vi "FGUDP.vi"(5 "Port":u16=5502, 7 "Remote Host":string="10.0.22.163", 8 "Error In":errorcluster, 10 "Data String In":string, 11 "UDP State":T1) -> (0 "error out":errorcluster, 2 "Data String Out":string)   [LabVIEW 2010, in "Flight Gear Data Custom Device.lvlib"]
uses:
  Flight Gear Data Custom Device.lvlib
  FlightGearState.ctl
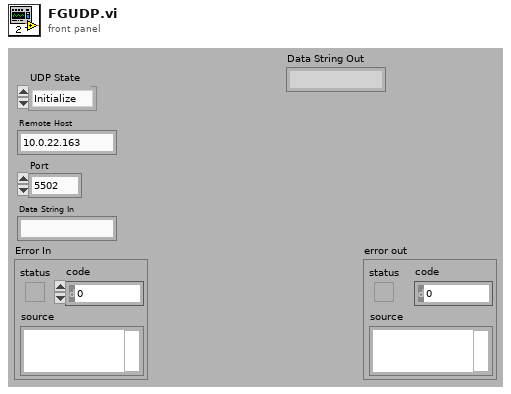
[diagram p1: front panel]
types:
  T1 = typedef "Flight Gear Data Custom Device.lvlib/FlightGearState.ctl" = enum16{"Initialize", "Read", "Write", "Close"}
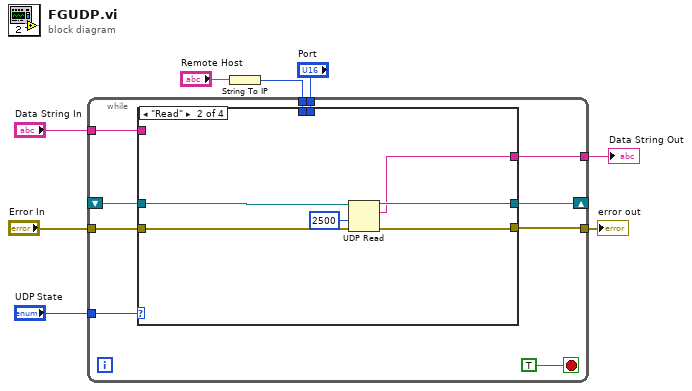
[diagram p0: block diagram]
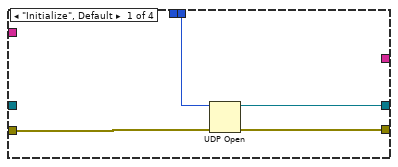
[diagram p2: hidden frame]
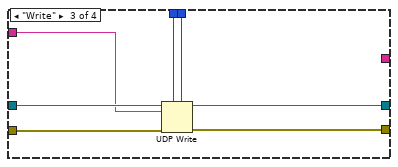
[diagram p3: hidden frame]
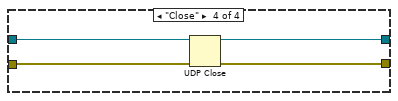
[diagram p4: hidden frame]
diagram:
  n1 = String To IP(1:"Remote Host") -> (0:w4:u32)
  n2 = while {
    tunnel: "UDP State" -> [w18]
    shift-right: [w14] -> _
    shift-left: _ -> [w13]
    tunnel: "Port" -> [w12]
    tunnel: w4 -> [w11]
    tunnel: "Data String In" -> [w10]
    tunnel: [w9] -> w1
    tunnel: "Error In" -> [w17]
    tunnel: [w16] -> w3
    stop <- TRUE stop-if-true
    n3 = case shown="\"Read\"" w18 {
      tunnel: w17 -> [w22 w27 w33 w36]
      tunnel: [w21 w26 w32 w37] -> w16
      tunnel: [w20 w25 w34 w38] -> w14
      tunnel: w13 -> [_ w28 w35 w39]
      tunnel: w12 -> [w19 _ w31 _]
      tunnel: w11 -> [_ _ w30 _]
      tunnel: w10 -> [_ _ w29 _]
      tunnel: [_ w24 _ _] -> w9
      frame "Initialize", Default {
        n4 = UDP Open(8:w22, 11:w19) -> (port=w20:refnum<k16>, 0:w21:errorcluster)  [unwired: 3 in, 1 out]
      }
      frame "Read" {
        n5 = UDP Read(connection ID=w28, timeout ms (25000)=2500, 8:w27) -> (data out=w24:string, error out=w26:errorcluster, 3:w25:refnum<k16>)  [unwired: 1 in, 2 out]
      }
      frame "Write" {
        n6 = UDP Write(address=w30, port or service name=w31, connection ID=w35, data in=w29, 8:w33) -> (error out=w32:errorcluster, 3:w34:refnum<k16>)  [unwired: 1 in]
      }
      frame "Close" {
        n7 = UDP Close(connection ID=w39, 8:w36) -> (connection ID out=w38:refnum<k16>, error out=w37:errorcluster)
      }
    }
  }
  "error out" <- w3
  "Data String Out" <- w1
